vi "FTW-Actor-OpeningHandshake.vi"(0 "FTW Actor Instance Type":refnum<class "FTW-Actor-Instance.lvclass">, 5 "Initialization Job Sequence":string, 7 "Actor Instance Configuration":string, 11 "error in":errorcluster) -> (4 "FTW Actor Instance":refnum<class "FTW-Actor-Instance.lvclass">, 6 "Incoming Request":refnum<event-registration>, 15 "error out":errorcluster)   [LabVIEW 2015, in "FTW-Actor-Instance.lvclass"]
uses:
  FTW-Actor-Instance.lvclass
  codegen/xnode/FTW-JSON-Fetch.xnode
  core/type/FTW-Type-JSON.ctl
  json/FTW-JSON-Type.ctl
  reflection/FTW-Reflection-Types.ctl
  lib/FTW-KernelFilepath.vi
  json/core/FTW-JSON-Core-LibraryReturnValue.vi
  codegen/xnode/json/fetch/FTW-JSON-Core-GetFlattenedValue.vi
  error/FTW-ERR-ThrowInvalidReferenceError.vi
  json/core/FTW-JSON-Core-Type.ctl
  json/core/FTW-JSON-Core-ElementType.vi
  json/FTW-JSON-SerializeAndDestroy.vi
  scheduler/FTW-Scheduler.lvclass
panel:
  # "Inputs"
  # "Outputs"
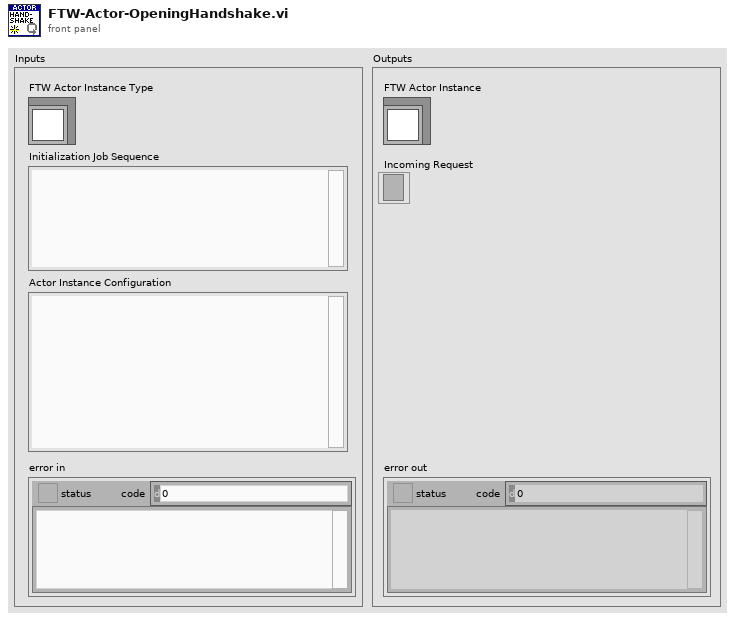
[diagram p1: front panel]
types:
  T1 = cluster{"Identity":string, "InboxAddress":string, "InboxConfiguration":string, "LauncherAddress":string, "HandshakeTimeout":i32}
  T2 = typedef "FTW-Type-JSON.ctl" = refnum<data-value>
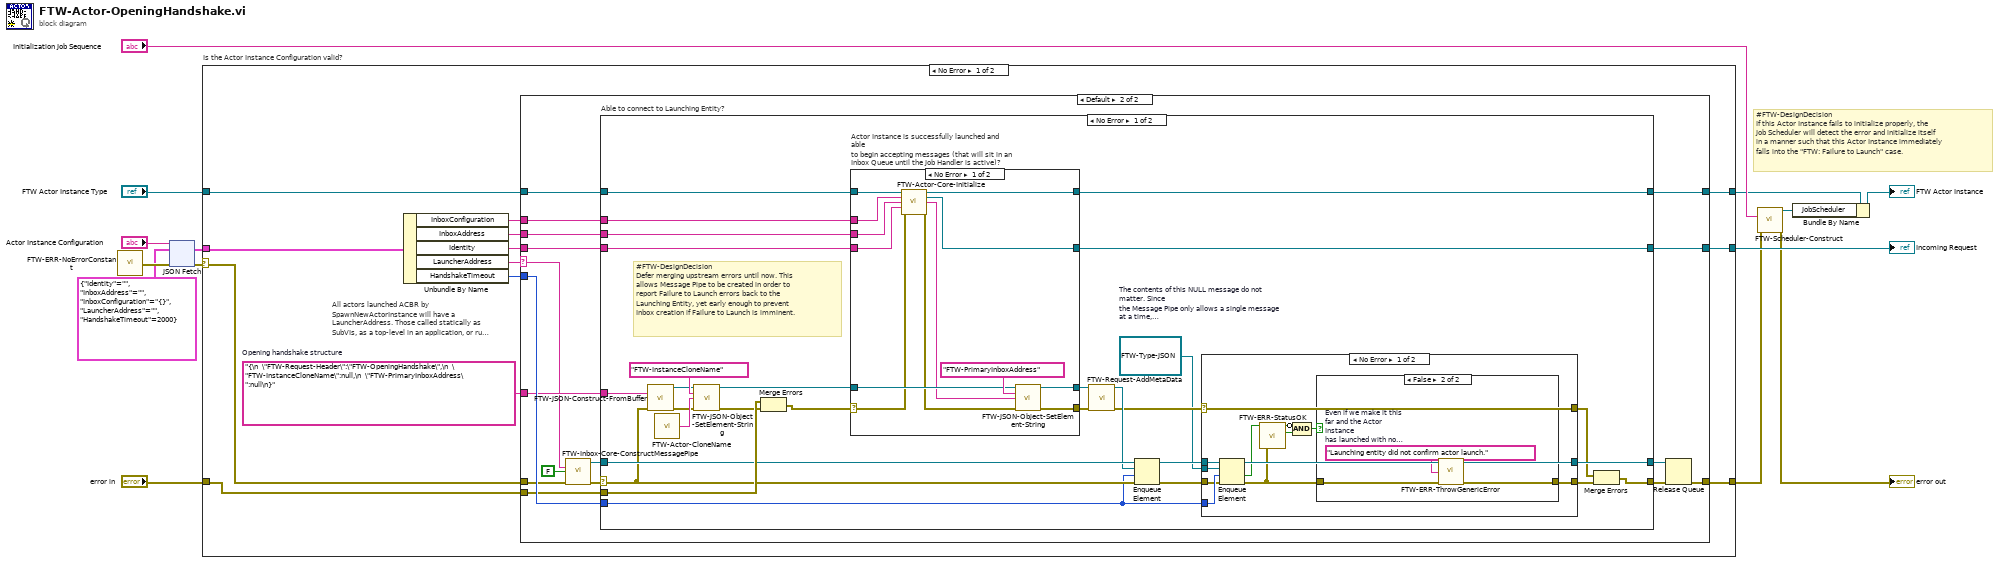
[diagram p0: block diagram]
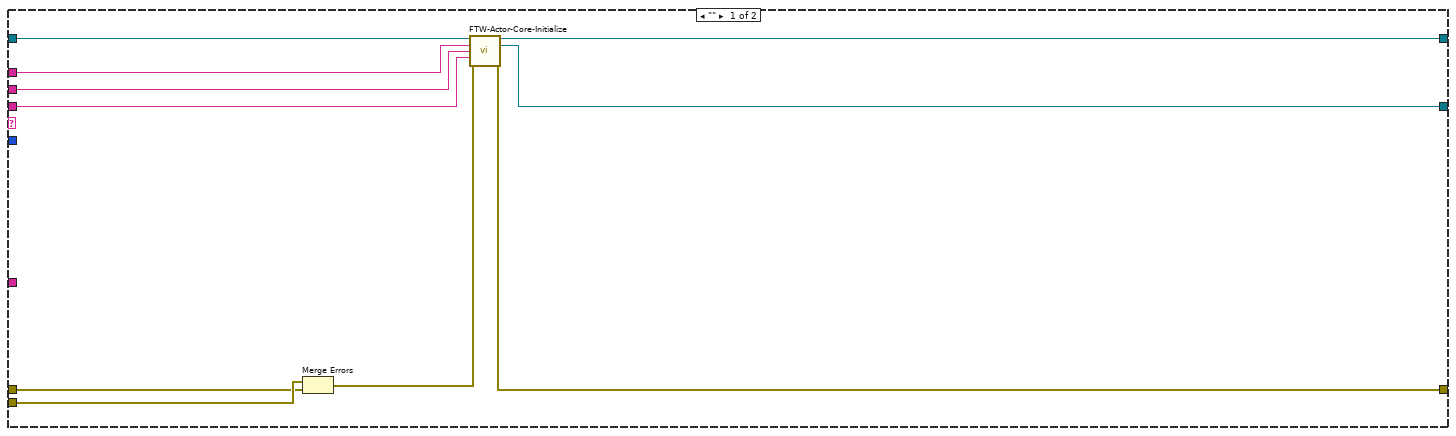
[diagram p2: hidden frame]
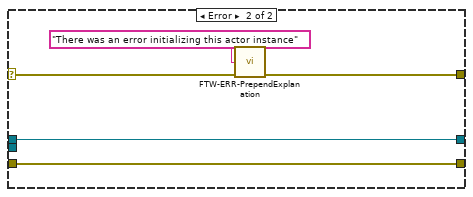
[diagram p4: hidden frame]
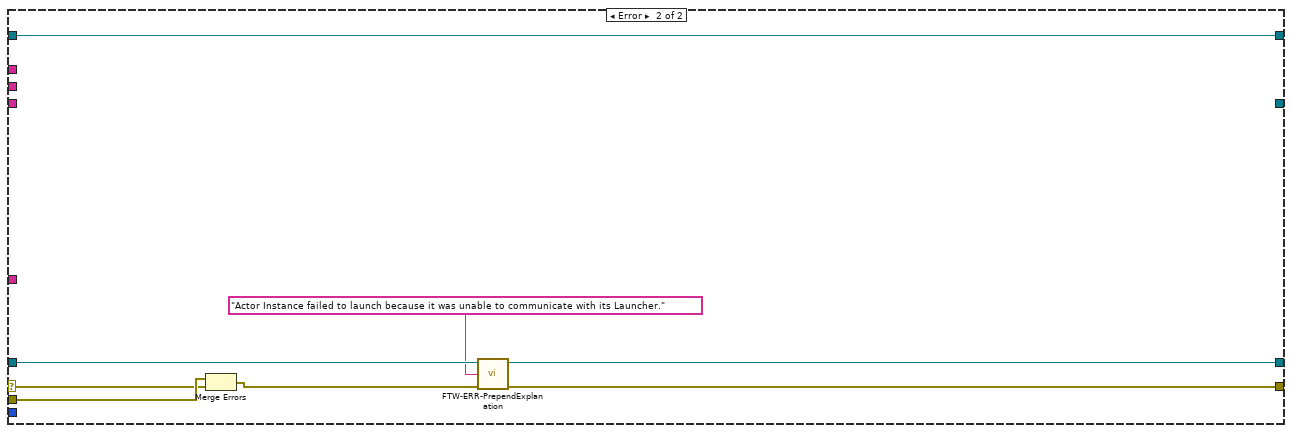
[diagram p6: hidden frame]
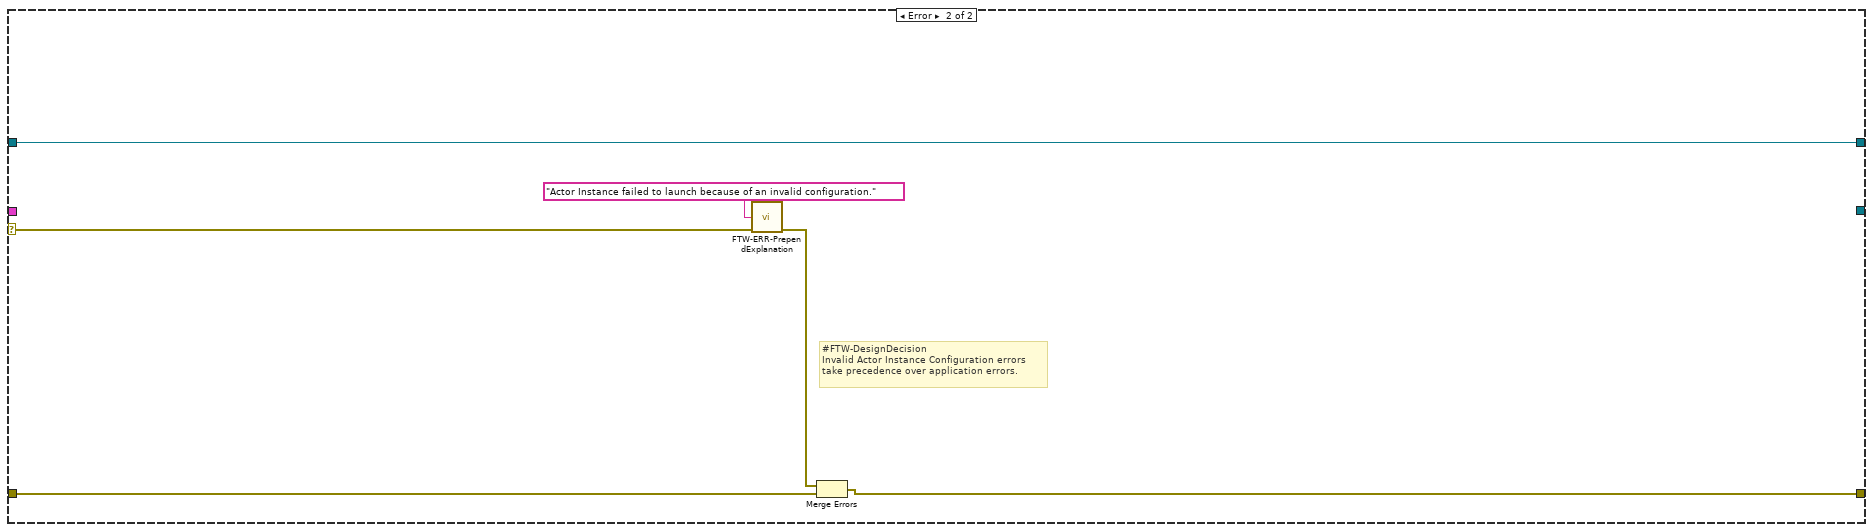
[diagram p7: hidden frame]
diagram:
  # "#FTW-DesignDecision\nIf this Actor Instance fails to initialize properly, the\nJob Scheduler will detect the error and initialize itself\nin a manner such that this Actor Instance immediately\nfalls into the \"FTW: Failure to Launch\" case."
  n1 = call "FTW-ERR-NoErrorConstant.vi"() -> ("no error"=w11:errorcluster)
  n2 = xnode "JSON Fetch"("JSON"="Actor Instance Configuration", "Element Type and Default Value"=T1 {"Identity"="", "InboxAddress"="", "InboxConfiguration"="{}", "LauncherAddress"="", "HandshakeTimeout"=2000}, "error in"=w11) -> ("Value"=w8:T1, "error out"=w10:errorcluster)  [unwired: 2 in, 2 out]
  n3 = case "Is the Actor Instance Configuration valid?" shown="No Error" w10 {
    selector: w10 -> [w17 w131]
    tunnel: "FTW Actor Instance Type" -> [w15 w132]
    tunnel: [w22 w127] -> w2
    tunnel: [w27 _] -> w13
    tunnel: [w26 w132] -> w4
    tunnel: w8 -> [w25 _]
    tunnel: "error in" -> [w16 w128]
    frame No Error {
      w19 = "{\n  \"FTW-Request-Header\":\"FTW-OpeningHandshake\",\n  \"FTW-InstanceCloneName\":null,\n  \"FTW-PrimaryInboxAddress\":null\n}"  # Opening handshake structure
      n4 = Unbundle By Name(w25) -> ("InboxConfiguration"=w20:string, "InboxAddress"=w24:string, "Identity"=w18:string, "LauncherAddress"=w21:string, "HandshakeTimeout"=w23:i32)
      n5 = case "All actors launched ACBR by SpawnNewActorInstance will have a LauncherAddress. Those called statically as SubVIs, as a top-level in an application, or run interactively in the IDE will not." shown="Default" w21 {
        selector: w21 -> [_ w43]
        tunnel: w15 -> [w37 w54]
        tunnel: [w32 w53] -> w27
        tunnel: [w36 w52] -> w26
        tunnel: w24 -> [w34 w51]
        tunnel: w23 -> [_ w50]
        tunnel: [w33 w45] -> w22
        tunnel: w16 -> [w30 w44]
        tunnel: w19 -> [_ w49]
        tunnel: w20 -> [w35 w48]
        tunnel: w18 -> [w31 w47]
        tunnel: w17 -> [w29 w42]
        frame "" {
          n6 = Merge Errors(w30, w29) -> (w28:errorcluster)
          n7 = call "FTW-Actor-Core-Initialize.vi"("FTW Actor Instance"=w37, "Inbox Configuration"=w35, "Primary Inbox Address"=w34, "Actor Identity"=w31, "error in"=w28) -> ("FTW Actor Instance out"=w36:refnum<class "FTW-Actor-Instance.lvclass">, "Incoming Request"=w32:refnum<event-registration>, "error out"=w33:errorcluster)  [unwired: 7 in, 1 out]
        }
        frame Default {
          n8 = call "FTW-Inbox-Core-ConstructMessagePipe.vi"("Actor Identity (empty to create unnamed actor)"=w43, "Is Primary?"=FALSE, "error in"=w42) -> ("Message Pipe"=w40:refnum<queue>, "error out"=w41:errorcluster)  [unwired: 10 in, 1 out]
          n9 = case "Able to connect to Launching Entity?" shown="No Error" w41 {
            selector: w41 -> [w62 w121]
            tunnel: w54 -> [w76 w125]
            tunnel: [w59 w124] -> w46
            tunnel: [w74 _] -> w53
            tunnel: [w73 w125] -> w52
            tunnel: w51 -> [w72 _]
            tunnel: w50 -> [w55 _]
            tunnel: w40 -> [w66 w126]
            tunnel: [w64 w126] -> w38
            tunnel: w49 -> [w77 _]
            tunnel: w48 -> [w75 _]
            tunnel: w47 -> [w71 _]
            tunnel: w44 -> [w70 w122]
            frame No Error {
              w56 = T2 refnum  # The contents of this NULL message do not matter. Since the Message Pipe only allows a single message at a time, the ability to enqueue a second message here is positive acknowledgement that the launcher received the first message. It's the synchronization that matters.
              # "#FTW-DesignDecision\nDefer merging upstream errors until now. This\nallows Message Pipe to be created in order to\nreport Failure to Launch errors back to the\nLaunching Entity, yet early enough to prevent\nInbox creation if Failure to Launch is imminent."
              n10 = call "FTW-JSON-Construct-FromBuffer.vi"("JSON String (UTF-8)"=w77, "error in"=w62) -> ("JSON"=w81:T2, "error out"=w80:errorcluster)  [unwired: 12 in]
              n11 = call "FTW-Actor-CloneName.vi"() -> ("Clone Name"=w83:string)  [unwired: 1 in]
              n12 = call "FTW-JSON-Object-SetElement-String.vi"("JSON"=w81, "Key"="FTW-InstanceCloneName", "Value"=w83, "error in"=w80) -> ("JSON out"=w79:T2, "error out"=w69:errorcluster)  [unwired: 10 in]
              n13 = Merge Errors(w70, w69) -> (w67:errorcluster)
              n14 = case "Actor Instance is successfully launched and able\nto begin accepting messages (that will sit in an\nInbox Queue until the Job Handler is active)?" shown="No Error" w67 {
                selector: w67 -> [w104 w117]
                tunnel: w79 -> [w115 w118]
                tunnel: [w114 w118] -> w78
                tunnel: w76 -> [w113 w119]
                tunnel: w75 -> [w112 _]
                tunnel: [w111 _] -> w74
                tunnel: [w108 w119] -> w73
                tunnel: w72 -> [w107 _]
                tunnel: w71 -> [w106 _]
                tunnel: [w105 w117] -> w68
                frame No Error {
                  n15 = call "FTW-Actor-Core-Initialize.vi"("FTW Actor Instance"=w113, "Inbox Configuration"=w112, "Primary Inbox Address"=w107, "Actor Identity"=w106, "error in"=w104) -> ("FTW Actor Instance out"=w108:refnum<class "FTW-Actor-Instance.lvclass">, "Incoming Request"=w111:refnum<event-registration>, "Resolved Primary Inbox Address"=w110:string, "error out"=w109:errorcluster)  [unwired: 7 in]
                  n16 = call "FTW-JSON-Object-SetElement-String.vi"("JSON"=w115, "Key"="FTW-PrimaryInboxAddress", "Value"=w110, "error in"=w109) -> ("JSON out"=w114:T2, "error out"=w105:errorcluster)  [unwired: 10 in]
                }
                frame Error {
                }
              }
              n17 = call "FTW-Request-AddMetaData.vi"("Response"=w78, "error in"=w68) -> ("Response out"=w58:T2, "error out"=w57:errorcluster)  [unwired: 12 in]
              n18 = Enqueue Element(queue=w66, element=w58, timeout in ms (-1)=w55, error in (no error)=w62) -> (queue out=w63:refnum<queue>, error out=w65:errorcluster)  [unwired: 1 out]
              n19 = case shown="No Error" w57 {
                selector: w57 -> [w93 w101]
                tunnel: [w94 w99] -> w60
                tunnel: w65 -> [w89 w99]
                tunnel: [w91 w103] -> w64
                tunnel: w55 -> [w90 _]
                tunnel: w63 -> [w92 w103]
                tunnel: [w93 w100] -> w61
                tunnel: w56 -> [w88 _]
                frame No Error {
                  n20 = Enqueue Element(queue=w92, element=w88, timeout in ms (-1)=w90, error in (no error)=w89) -> (queue out=w91:refnum<queue>, timed out?=w87:bool, error out=w84:errorcluster)
                  n21 = call "FTW-ERR-StatusOK.vi"("error to check"=w84) -> ("Status OK?"=w86:bool)
                  n22 = Compound Arithmetic op=AND(invert w87, w86) -> (w85:bool)
                  n23 = case shown="False" w85 {
                    tunnel: [w95 w98] -> w94
                    tunnel: w84 -> [w95 w96]
                    frame True {
                      # "Success."
                    }
                    frame False {
                      w97 = "Launching entity did not confirm actor launch."  # Even if we make it this far and the Actor Instance has launched with no error, we treat the lack of response from the Launcher as a fatal error, such that this Actor Instance does not exist as a renegade.
                      n24 = call "FTW-ERR-ThrowGenericError.vi"("Error Message"=w97, "error in"=w96) -> ("error out"=w98:errorcluster)  [unwired: 13 in]
                    }
                  }
                }
                frame Error {
                  n25 = call "FTW-ERR-PrependExplanation.vi"("Exception Information"="There was an error initializing this actor instance", "error in"=w101) -> ("error out"=w100:errorcluster)  [unwired: 13 in]
                }
              }
              n26 = Merge Errors(w61, w60) -> (w59:errorcluster)
            }
            frame Error {
              n27 = Merge Errors(w122, w121) -> (w120:errorcluster)
              n28 = call "FTW-ERR-PrependExplanation.vi"("Exception Information"="Actor Instance failed to launch because it was unable to communicate with its Launcher." ("Error Message"), "error in"=w120) -> ("error out"=w124:errorcluster)  [unwired: 13 in]
            }
          }
          n29 = Release Queue(queue=w38, error in (no error)=w46) -> (error out=w45:errorcluster)  [unwired: 1 in, 2 out]
        }
      }
    }
    frame Error {
      # "#FTW-DesignDecision\nInvalid Actor Instance Configuration errors\ntake precedence over application errors."
      n30 = call "FTW-ERR-PrependExplanation.vi"("Exception Information"="Actor Instance failed to launch because of an invalid configuration." ("Error Message"), "error in"=w131) -> ("error out"=w130:errorcluster)  [unwired: 13 in]
      n31 = Merge Errors(w130, w128) -> (w127:errorcluster)
    }
  }
  "Incoming Request" <- w13
  n32 = call "FTW-Scheduler-Construct.vi"("Initial Job Sequence"="Initialization Job Sequence", "error in"=w2) -> ("FTW Job Scheduler"=w1:refnum<class "FTW-Scheduler.lvclass">, "error out"=→"error out":errorcluster)  [unwired: 12 in]
  n33 = Bundle By Name(cluster=w4, "JobScheduler"=w1) -> (→"FTW Actor Instance":refnum<class "FTW-Actor-Instance.lvclass">)
